vi "Log On.vi"(8 "error in":errorcluster, 10 "Log On":bool, 11 "Base Software in":refnum<class "Base Software.lvclass">) -> (0 "error out":errorcluster, 3 "Base Software out":refnum<class "Base Software.lvclass">)   [LabVIEW 2019, in "Base Software.lvlib" / "Main.lvlib" / "Base Software.lvclass"]
uses:
  Project/Base Software.lvclass
  Project/Base Software.lvclass/Base Software.ctl
  Accessors/StateMachine/Write Logged_On.vi
  Accessors/Indicators/Write Witness.vi
  Accessors/Indicators/Write Operator.vi
  Accessors/Buttons/Login.vi
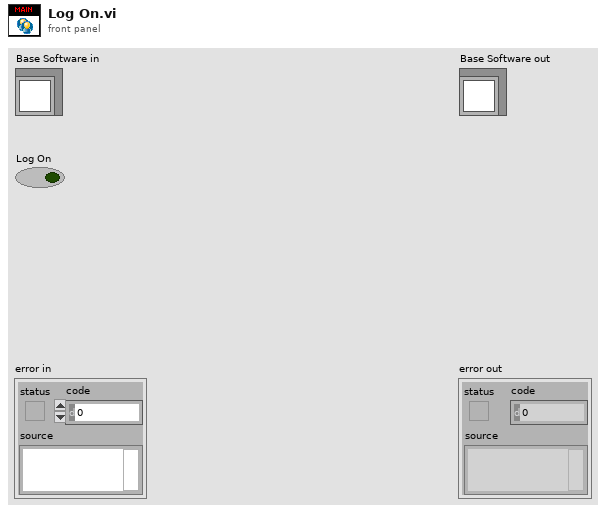
[diagram p1: front panel]
types:
  T1 = typedef "Engine.lvlibp/Engine.lvclass/System Status.ctl" = enum16{"Logged Off", "UUT_Info_Missing", "Idle", "Error", "Warning", "Loading", "Config", "Manual", "Automation", "Report_View", "Previous"}
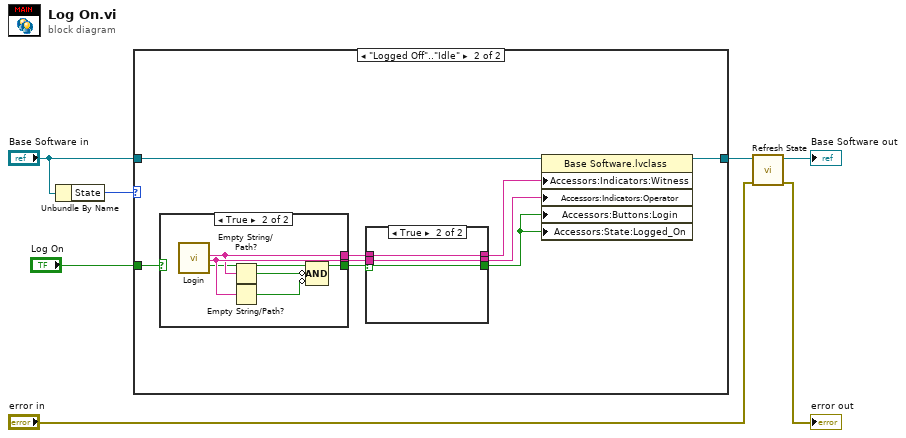
[diagram p0: block diagram]
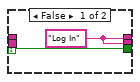
[diagram p4: hidden frame]
diagram:
  n1 = Unbundle By Name("Base Software in") -> ("State"=w5:T1)
  n2 = case shown="\"Logged Off\"..\"Idle\"" w5 {
    tunnel: "Base Software in" -> [w8 w17]
    tunnel: [w8 w10] -> w4
    tunnel: "Log On" -> [_ w11]
    frame Default {
      # "System is running, changing users is not allowed"
    }
    frame "Logged Off".."Idle" {
      n3 = case shown="True" w11 {
        selector: w11 -> [w18 _]
        tunnel: [_ w24] -> w14
        tunnel: [_ w23] -> w13
        tunnel: [w18 w21] -> w12
        frame False {
        }
        frame True {
          n4 = call "Login"() -> ("Test Witness"=w23:string, "Test Operator"=w24:string, "OK"=w22:bool)  [unwired: 16 in, 1 out]
          n5 = Empty String/Path?(string/path=w23) -> (empty?=w20:bool)
          n6 = Empty String/Path?(string/path=w24) -> (empty?=w19:bool)
          n7 = Compound Arithmetic op=AND(w22, invert w20, invert w19) -> (w21:bool)
        }
      }
      n8 = case shown="True" w12 {
        selector: w12 -> [w25 w27]
        tunnel: w13 -> [_ w29]
        tunnel: w14 -> [_ w28]
        tunnel: [w26 w29] -> w16
        tunnel: [w26 w28] -> w15
        tunnel: [w25 w27] -> w9
        frame False {
          w26 = "Log In" ("Test Witness")
        }
        frame True {
        }
      }
      n9 = property class="Base Software.lvclass"(reference=w17, "Accessors:Indicators:Witness"=w16, "Accessors:Indicators:Operator"=w15, "Accessors:Buttons:Login"=w9, "Accessors:State:Logged_On"=w9) -> (reference out=w10:refnum<class "Base Software.lvclass">)  [unwired: 1 in, 1 out]
    }
  }
  n10 = call "Refresh State.vi"("error in"="error in", "Base Software in"=w4) -> ("error out"=→"error out":errorcluster, "Base Software out"=→"Base Software out":refnum<class "Base Software.lvclass">)  [unwired: 8 in]
